vi "Initialize.vi"(8 "error in (no error)":errorcluster, 11 "ASIA Pump C Settings in":T1 {"channel" min=-1 max=1 step=1; "ASIA Pump #" min=0 step=1}) -> (0 "error out":errorcluster, 1 "Initialized":bool, 2 "No Pump Connected":bool=TRUE, 3 "ASIA Pump C Settings out":T1)   [LabVIEW 2018, in "ASIA Pump.lvlib"]
uses:
  ASIA Pump.lvlib
  Pump Settings.ctl
panel:
  out "appended path":path
  out "path out 2":path
  out "path out":path
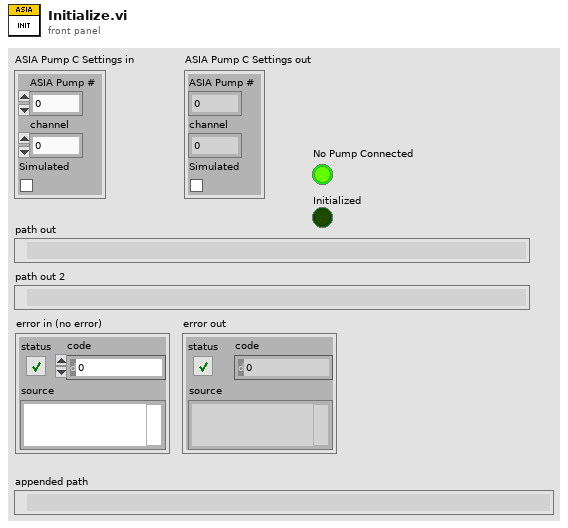
[diagram p1: front panel]
types:
  T1 = typedef "ASIA Pump.lvlib/Pump Settings.ctl" = cluster{"ASIA Pump #":i32, "channel":i32, "Simulated":bool}
  T2 = enum16{"Error", "Uninitialised", "Initialising", "Idle", "Filling", "Full", "Emptying", "Empty", "Pumping", "Default"}
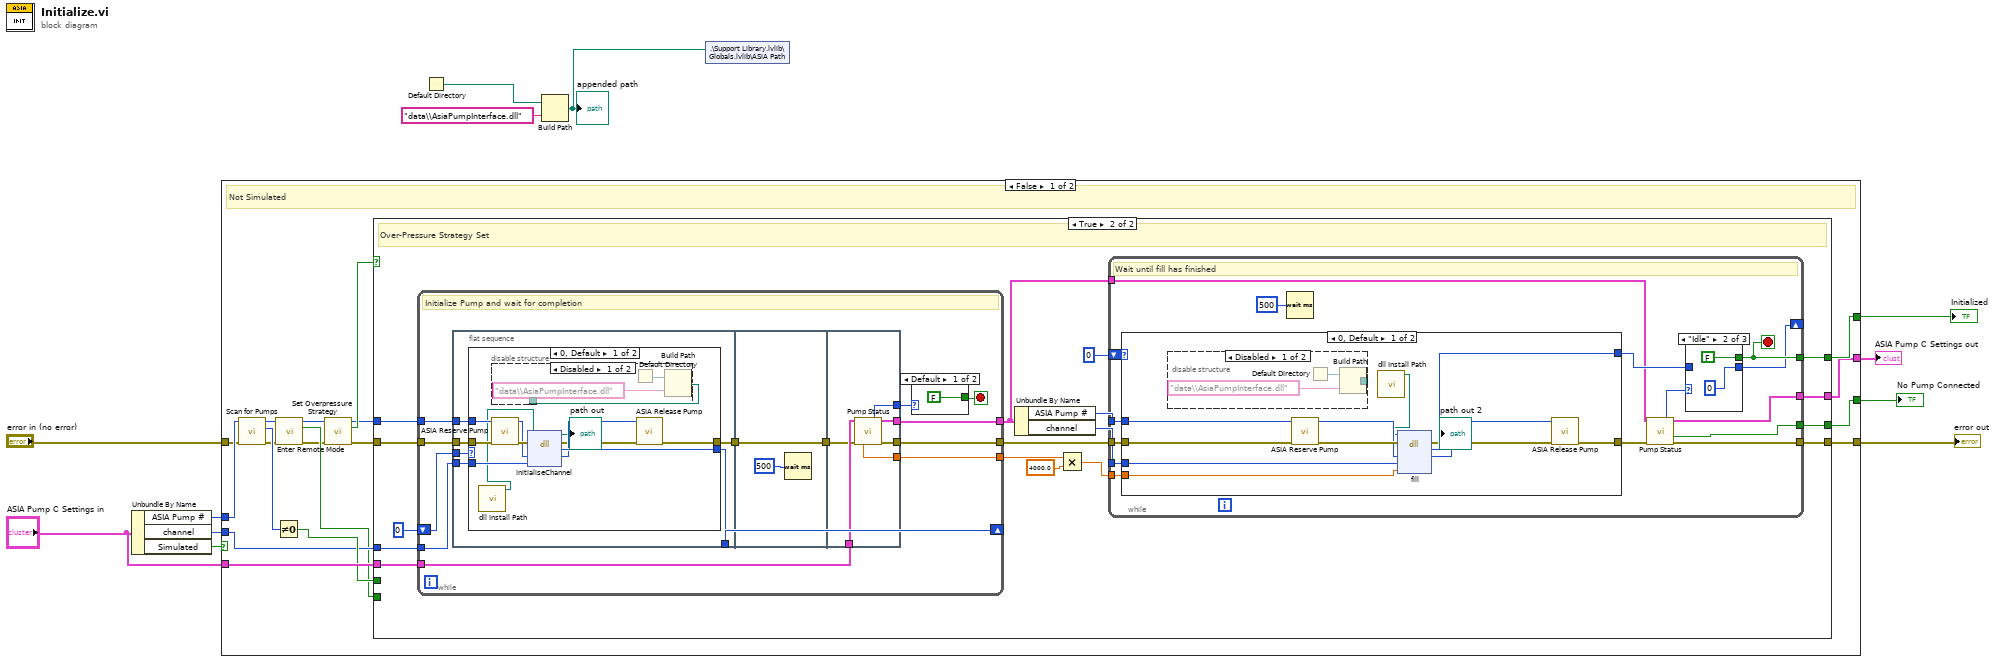
[diagram p0: block diagram]
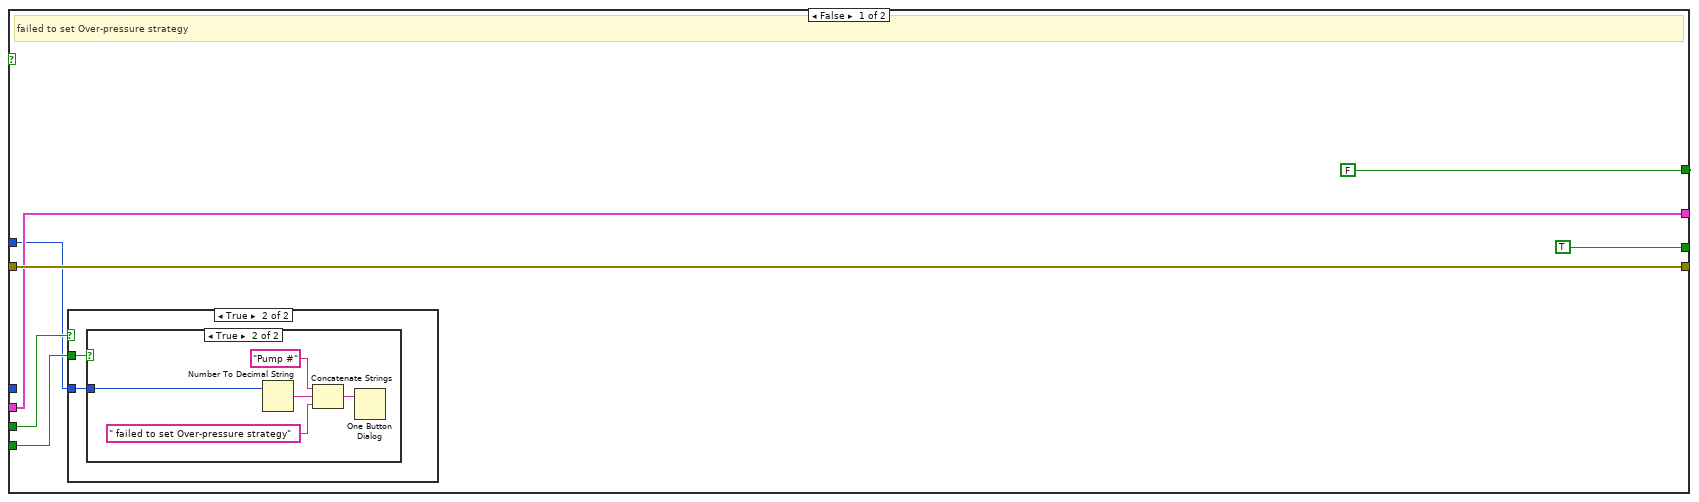
[diagram p2: hidden frame]
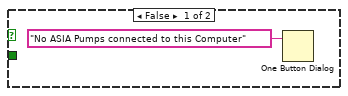
[diagram p3: hidden frame]
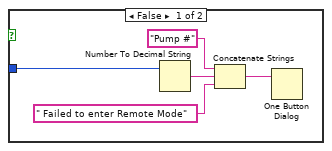
[diagram p4: hidden frame]
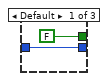
[diagram p7: hidden frame]
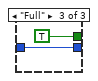
[diagram p8: hidden frame]
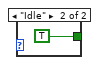
[diagram p11: hidden frame]
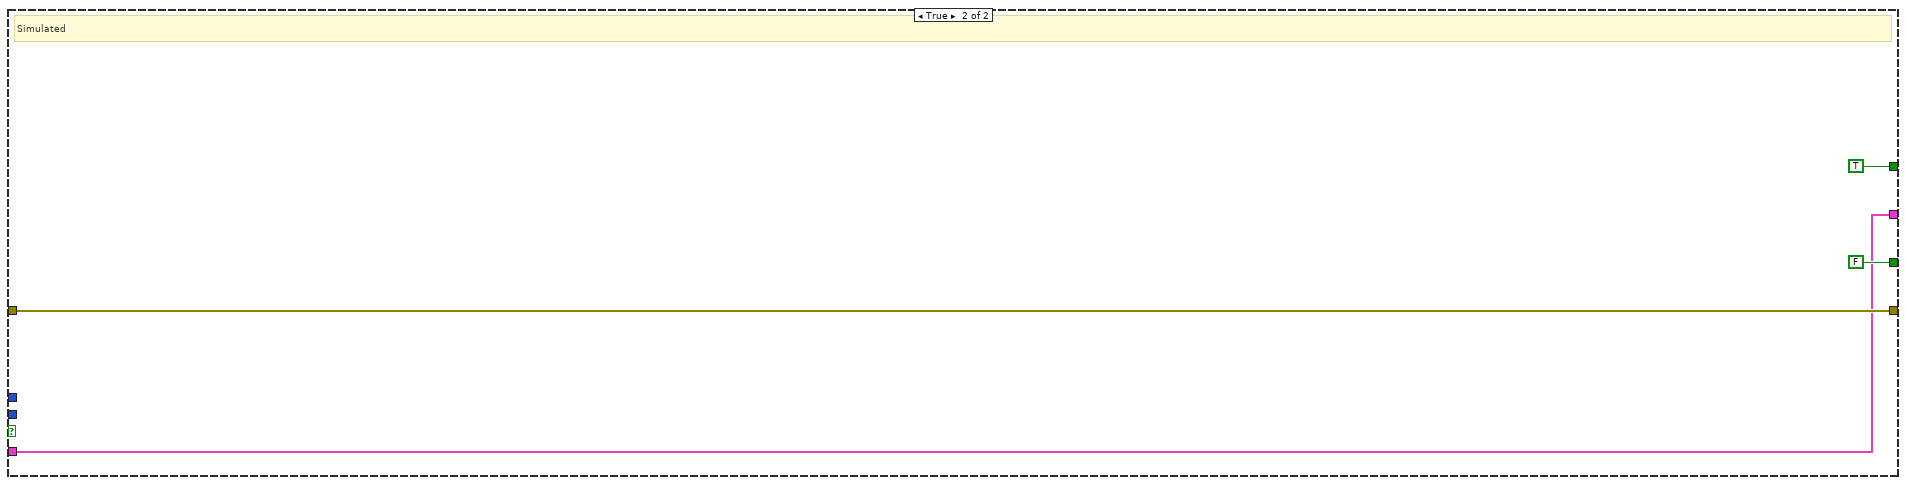
[diagram p12: hidden frame]
diagram:
  n1 = Unbundle By Name("ASIA Pump C Settings in") -> ("ASIA Pump #"=w4:i32, "channel"=w6:i32, "Simulated"=w5:bool)
  n2 = case shown="False" w5 {
    tunnel: "error in (no error)" -> [w22 w153]
    tunnel: [w30 w153] -> w12
    tunnel: w6 -> [w24 _]
    tunnel: [w29 FALSE] -> w11
    tunnel: "ASIA Pump C Settings in" -> [w28 w150]
    tunnel: [w27 TRUE] -> w10
    tunnel: [w25 w150] -> w9
    tunnel: w4 -> [w23 _]
    frame False {
      # "Not Simulated"
      n3 = call "Scan for Pumps.vi"("error in (no error)"=w22, "ASIA Pump # In"=w23) -> ("error out"=w18:errorcluster, "pumpCnt"=w21:u32, "ASIA Pump # Out"=w19:i32)  [unwired: 7 in]
      n4 = Not Equal To 0?(x=w21) -> (x != 0?=w26:bool)
      n5 = call "Enter Remote Mode.vi"("error in (no error)"=w18, "ASIA Pump #"=w19) -> ("error out"=w16:errorcluster, "Completed"=w20:bool, "ASIA Pump #"=w17:i32)  [unwired: 7 in]
      n6 = call "Set Overpressure Strategy.vi"("error in (no error)"=w16, "ASIA Pump # In"=w17) -> ("error out"=w14:errorcluster, "strategySet"=w15:bool, "ASIA Pump # Out"=w13:i32)  [unwired: 7 in]
      n7 = case shown="True" w15 {
        tunnel: w14 -> [w36 w66]
        tunnel: [TRUE w54] -> w29
        tunnel: [w36 w55] -> w30
        tunnel: w13 -> [w31 w63]
        tunnel: w28 -> [w32 w64]
        tunnel: [FALSE w53] -> w27
        tunnel: w26 -> [w34 _]
        tunnel: w20 -> [w33 _]
        tunnel: w24 -> [_ w62]
        tunnel: [w32 w51] -> w25
        frame False {
          # "failed to set Over-pressure strategy"
          n8 = case shown="True" w34 {
            tunnel: w33 -> [_ w40]
            tunnel: w31 -> [_ w39]
            frame False {
              n9 = One Button Dialog(message="No ASIA Pumps connected to this Computer") -> ()  [unwired: 1 in, 1 out]
            }
            frame True {
              n10 = case shown="True" w40 {
                tunnel: w39 -> [w41 w46]
                frame False {
                  n11 = Number To Decimal String(number=w41) -> (decimal integer string=w44:string)  [unwired: 1 in]
                  n12 = Concatenate Strings("Pump #" ("string"), w44, " Failed to enter Remote Mode" ("message")) -> (w45:string)
                  n13 = One Button Dialog(message=w45) -> ()  [unwired: 1 in, 1 out]
                }
                frame True {
                  n14 = Number To Decimal String(number=w46) -> (decimal integer string=w49:string)  [unwired: 1 in]
                  n15 = Concatenate Strings("Pump #" ("string"), w49, " failed to set Over-pressure strategy" ("message")) -> (w50:string)
                  n16 = One Button Dialog(message=w50) -> ()  [unwired: 1 in, 1 out]
                }
              }
            }
          }
        }
        frame True {
          # "Over-Pressure Strategy Set"
          n17 = while {
            tunnel: [w110] -> w57
            tunnel: w66 -> [w116]
            tunnel: [w109] -> w56
            tunnel: w63 -> [w115]
            tunnel: w62 -> [w114]
            tunnel: w64 -> [w111]
            tunnel: [w107] -> w61
            shift-right: [w106] -> _
            shift-left: u8 0 ("Bool") -> [w105]
            stop <- w117 stop-if-true
            # "Initialize Pump and wait for completion"
            n18 = flat-sequence {
              tunnel: w116 -> [w123]
              tunnel: w115 -> [w121]
              tunnel: w114 -> [w120]
              tunnel: [w122] -> w113
              tunnel: [w119] -> w106
              tunnel: w105 -> [w118]
              tunnel: w113 -> [w141]
              tunnel: [w141] -> w112
              tunnel: w112 -> [w146]
              tunnel: w111 -> [w147]
              tunnel: [w145] -> w110
              tunnel: [w144] -> w109
              tunnel: [w143] -> w108
              tunnel: [w142] -> w107
              frame #0 {
                n19 = case shown="0, Default" w118 {
                  selector: w118 -> [_ w138]
                  tunnel: w123 -> [w132 w139]
                  tunnel: [w126 w139] -> w122
                  tunnel: w121 -> [w130 _]
                  tunnel: w120 -> [w134 _]
                  tunnel: [w133 w138] -> w119
                  frame 0, Default {
                    n20 = call "dll Install Path.vi"() -> ("system directory"=w125:path)  [unwired: 11 in]
                    n21 = call "ASIA Reserve Pump.vi"("error in (no error)"=w132, "ASIA Pump # In"=w130) -> ("error out"=w131:errorcluster, "ASIA Pump # Out"=w129:i32)  [unwired: 8 in]
                    n22 = disable-structure shown="Disabled" {
                      disable-tunnel: [w135 _] -> _
                      frame Disabled {
                        n23 = Default Directory() -> (w136:path)
                        n24 = Build Path(base path=w136, name or relative path="data\\AsiaPumpInterface.dll") -> (appended path=w135:path)
                      }
                      frame Enabled {
                      }
                    }
                    n25 = dll-call lib="C:/Program Files (x86)/Pfizer/FAST/data/AsiaPumpInterface.dll" fn="initialiseChannel"(path in=w125, error in=w131, "pumpNum"=w129, "channel"=w134) -> (path out=→"path out":path, error out=w127:errorcluster, "Bool"=w133:u8, "pumpNum"=w128:u32)  [unwired: 2 in]
                    n26 = call "ASIA Release Pump.vi"("error in (no error)"=w127, "pumpNum"=w128) -> ("error out"=w126:errorcluster)  [unwired: 8 in, 1 out]
                  }
                  frame 1 {
                  }
                }
              }
              frame #1 {
                n27 = Wait (ms)(milliseconds to wait=u32 500) -> ()  [unwired: 1 out]
              }
              frame #2 {
                n28 = call "Pump Status.vi"("ASIA Pump C Settings in"=w147, "error in (no error)"=w146) -> ("PumpStatusCode"=w143:T2, "ASIA Pump C Settings out"=w144:T1, "syringeSize (ml)"=w142:sgl, "error out"=w145:errorcluster)  [unwired: 5 in, 5 out]
              }
            }
            n29 = case shown="Default" w108 {
              tunnel: [FALSE TRUE] -> w117
              frame Default {
              }
              frame "Idle" {
              }
            }
          }
          n30 = Unbundle By Name(w56) -> ("ASIA Pump #"=w59:i32, "channel"=w58:i32)
          n31 = Multiply(x=w61, y=4000.0) -> (x*y=w60:dbl)
          n32 = while {
            tunnel: [w72] -> w55
            tunnel: w56 -> [w71]
            tunnel: w57 -> [w81]
            tunnel: w59 -> [w80]
            tunnel: w58 -> [w79]
            tunnel: w60 -> [w78]
            tunnel: [w77] -> w53
            tunnel: [w68] -> w54
            shift-right: [w74] -> _
            shift-left: u8 0 ("Bool") -> [w76]
            tunnel: [w69] -> w51
            stop <- w77 stop-if-true
            # "Wait until fill has finished"
            n33 = case shown="0, Default" w76 {
              selector: w76 -> [_ w97]
              tunnel: w81 -> [w89 w98]
              tunnel: w80 -> [w90 _]
              tunnel: w79 -> [w93 _]
              tunnel: w78 -> [w92 _]
              tunnel: [w84 w98] -> w73
              tunnel: [w91 w97] -> w75
              frame 0, Default {
                n34 = disable-structure shown="Disabled" {
                  disable-tunnel: [w94 _] -> _
                  frame Disabled {
                    n35 = Default Directory() -> (w95:path)
                    n36 = Build Path(base path=w95, name or relative path="data\\AsiaPumpInterface.dll") -> (appended path=w94:path)
                  }
                  frame Enabled {
                  }
                }
                n37 = call "ASIA Reserve Pump.vi"("error in (no error)"=w89, "ASIA Pump # In"=w90) -> ("error out"=w88:errorcluster, "ASIA Pump # Out"=w87:i32)  [unwired: 8 in]
                n38 = call "dll Install Path.vi"() -> ("system directory"=w83:path)  [unwired: 11 in]
                n39 = dll-call lib="C:/Program Files (x86)/Pfizer/FAST/data/AsiaPumpInterface.dll" fn="fill"(path in=w83, error in=w88, "pumpNum"=w87, "channel"=w93, "rate"=w92) -> (error out=w86:errorcluster, "Bool"=w91:u8, "pumpNum"=w85:u32)  [unwired: 3 in, 1 out]
                n40 = call "ASIA Release Pump.vi"("error in (no error)"=w86, "pumpNum"=w85) -> ("error out"=w84:errorcluster)  [unwired: 8 in, 1 out]
              }
              frame 1 {
              }
            }
            n41 = Wait (ms)(milliseconds to wait=u32 500) -> ()  [unwired: 1 out]
            n42 = call "Pump Status.vi"("ASIA Pump C Settings in"=w71, "error in (no error)"=w73) -> ("PumpStatusCode"=w70:T2, "ASIA Pump C Settings out"=w69:T1, "Connection Error"=w68:bool, "error out"=w72:errorcluster)  [unwired: 5 in, 5 out]
            n43 = case shown="\"Idle\"" w70 {
              tunnel: [FALSE FALSE TRUE] -> w77
              tunnel: w75 -> [w99 _ w103]
              tunnel: [w99 0 w103] -> w74
              frame Default {
              }
              frame "Idle" {
              }
              frame "Full" {
              }
            }
          }
        }
      }
    }
    frame True {
      # "Simulated"
    }
  }
  "error out" <- w12
  "ASIA Pump C Settings out" <- w9
  "No Pump Connected" <- w11
  "Initialized" <- w10
  n44 = Default Directory() -> (w1:path)
  n45 = Build Path(base path=w1, name or relative path="data\\AsiaPumpInterface.dll") -> (appended path=w2:path)
  "appended path" <- w2
  n46 = shared-variable ".\\Support Library.lvlib\\Globals.lvlib\\ASiA Path"(w2) -> ()  [unwired: 1 in, 1 out]
